vi "filter_.vi"(7 "滤波方法":enum16{"Butterworth", "Chebyshev"}(ring), 8 "阶数":i32(slide) min=0 max=5 step=1 scale=0.0..5.0, 9 "截止频率":dbl(slide) scale=0.0..200.0, 10 "采样频率 (fs)":dbl, 11 "输入信号":dbl[](graph)) -> (3 "输出信号":dbl[](graph))   [LabVIEW 2022 SP3]
uses:
  <vilib>/Analysis/3filter.llb/Filter Passband Type.ctl
  <vilib>/Analysis/3filter.llb/Butterworth Filter (DBL).vi
  <vilib>/Analysis/3filter.llb/Chebyshev Filter (DBL).vi
  <vilib>/Analysis/NI_AALBase.lvlib
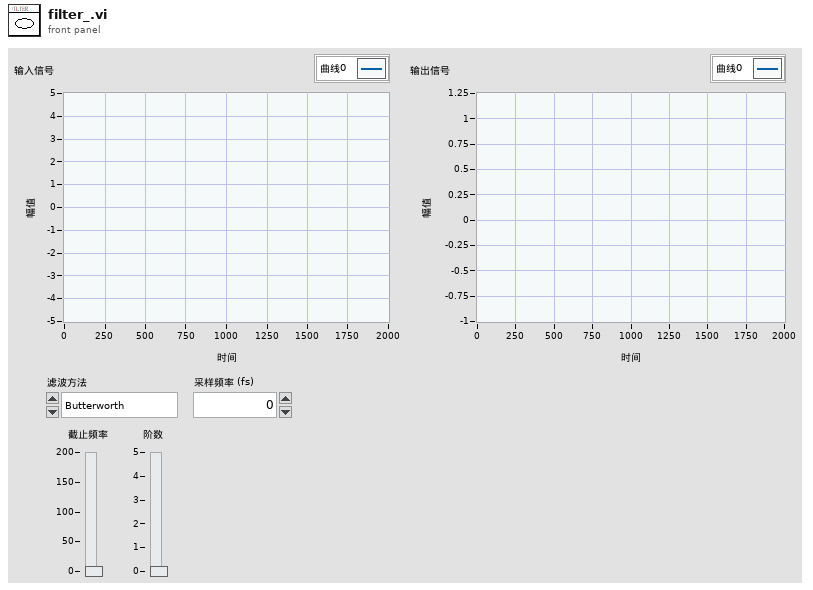
[diagram p1: front panel]
types:
  T1 = typedef "NI_AALBase.lvlib/Filter Passband Type.ctl" = enum32{"Lowpass", "Highpass", "Bandpass", "Bandstop"}
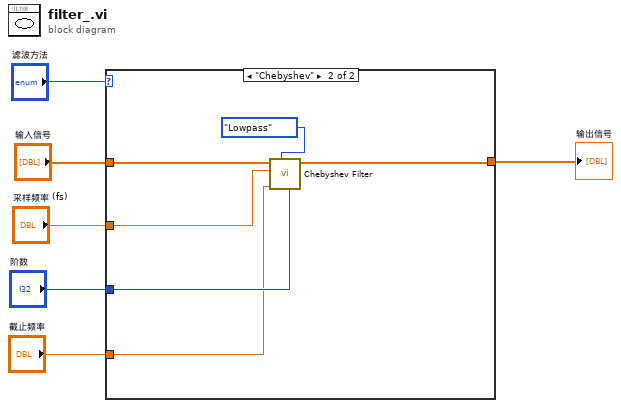
[diagram p0: block diagram]
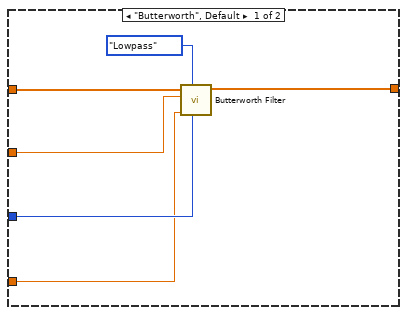
[diagram p2: hidden frame]
diagram:
  n1 = case shown="\"Chebyshev\"" "滤波方法" {
    tunnel: "输入信号" -> [w12 w18]
    tunnel: [w11 w17] -> w4
    tunnel: "采样频率 (fs)" -> [w10 w16]
    tunnel: "阶数" -> [w9 w15]
    tunnel: "截止频率" -> [w8 w14]
    frame "Butterworth", Default {
      n2 = call-poly <vilib>:"Butterworth Filter.vi"("order"=w9, "filter type"=Filter_Passband_Type."Lowpass", "low cutoff freq: fl"=w8, "sampling freq: fs"=w10, "X"=w12) -> ("Filtered X"=w11:dbl[])  [unwired: 3 in, 1 out]
    }
    frame "Chebyshev" {
      n3 = call-poly <vilib>:"Chebyshev Filter.vi"("order"=w15, "filter type"=Filter_Passband_Type."Lowpass", "low cutoff freq: fl"=w14, "sampling freq: fs"=w16, "X"=w18) -> ("Filtered X"=w17:dbl[])  [unwired: 5 in, 1 out]
    }
  }
  "输出信号" <- w4
